vi "Find Average Center.vi"(5 "Position":i32, 7 "Tray Number":i32, 9 "XYZTheta":dbl[](array[numeric]), 11 "Gantry In":refnum<k24>) -> (1 "XYZTheta":dbl[](array[numeric]) format="%.6g", 3 "Gantry Out":refnum<k24>)   [LabVIEW 2019, in "Component Tray.lvclass"]
uses:
  Component Tray.lvclass
  Find Component.ctl
  Controller/Camera/Machine Vision.ctl
  C:/Program Files (x86)/Aerotech/A3200/LabVIEW/2010/Bin/Aerotech.A3200.dll
  Program Files (x86)/Aerotech/A3200/LabVIEW/2010/Bin/Aerotech.A3200.dll
  Controller/Camera/Image processing.ctl
  Controller/Camera/Camera settings.ctl
  Controller/Camera/Material.ctl
  Controller/Camera/Edmund Optics/Edmund Optics.lvclass
  C:/Users/HEP/Documents/Aerotech gantry/UCSB-Gantry-master-main/V5/Classes/Controller/Camera/Camera.lvclass
  Controller/Motion/A3200/A3200.lvclass
  Controller/Camera/Camera.lvclass
panel:
  in  "Material":T1
  out "All fiducials recorded":bool
  in  "Override presets":bool
  in  "Camera settings":T2={"Gamma"=1.6, "Gain"=0, "Sharpness"=0, "Contrast"=0.0, "Exposure"=0.0078125} {"Exposure" min=0.000244140625 max=0.5 scale=0.0002..0.5; "Contrast" min=0.0 max=1.0 scale=0.001..1.0; "Sharpness" min=0 max=2 step=1 scale=0.0..2.0; "Gain" min=0 max=100 step=1 scale=0.1..100.0; "Gamma" min=0.01 max=10.0 scale=0.01..10.0}
  in  "Image processing":T3={"Brightness"=128.0, "Contrast"=45.0, "Gamma"=1.0471123} {"Brightness" scale=0.0..400.0; "Contrast" scale=0.0..90.0; "Gamma" scale=0.005..5.0}
  in  "Machine Vision":T4
  out "Gantry":dbl[](array[numeric])
  out "Sum":dbl[](array[numeric])
  out "BR XY":dbl[](array[numeric]) format="%.6g"
  out "TR XY":dbl[](array[numeric]) format="%.6g"
  out "BL XY":dbl[](array[numeric]) format="%.6g"
  out "TL XY":dbl[](array[numeric]) format="%.6g"
  in  "Record Top Right":bool
  in  "Record Bottom Right":bool
  in  "Record Bottom Left":bool
  in  "Record Top Left":bool
  in  "Go to Bottom Right":bool
  in  "Go to Top Right":bool
  in  "Go to Bottom Left":bool
  in  "Go to Top Left":bool
  in  "Joystick":bool
  out "Camera":dbl[](array[numeric])
  in  "Go to Center":bool
  in  "Component":T5
  in  "Stop Program":bool
  out "Image":T6(plugin-control)
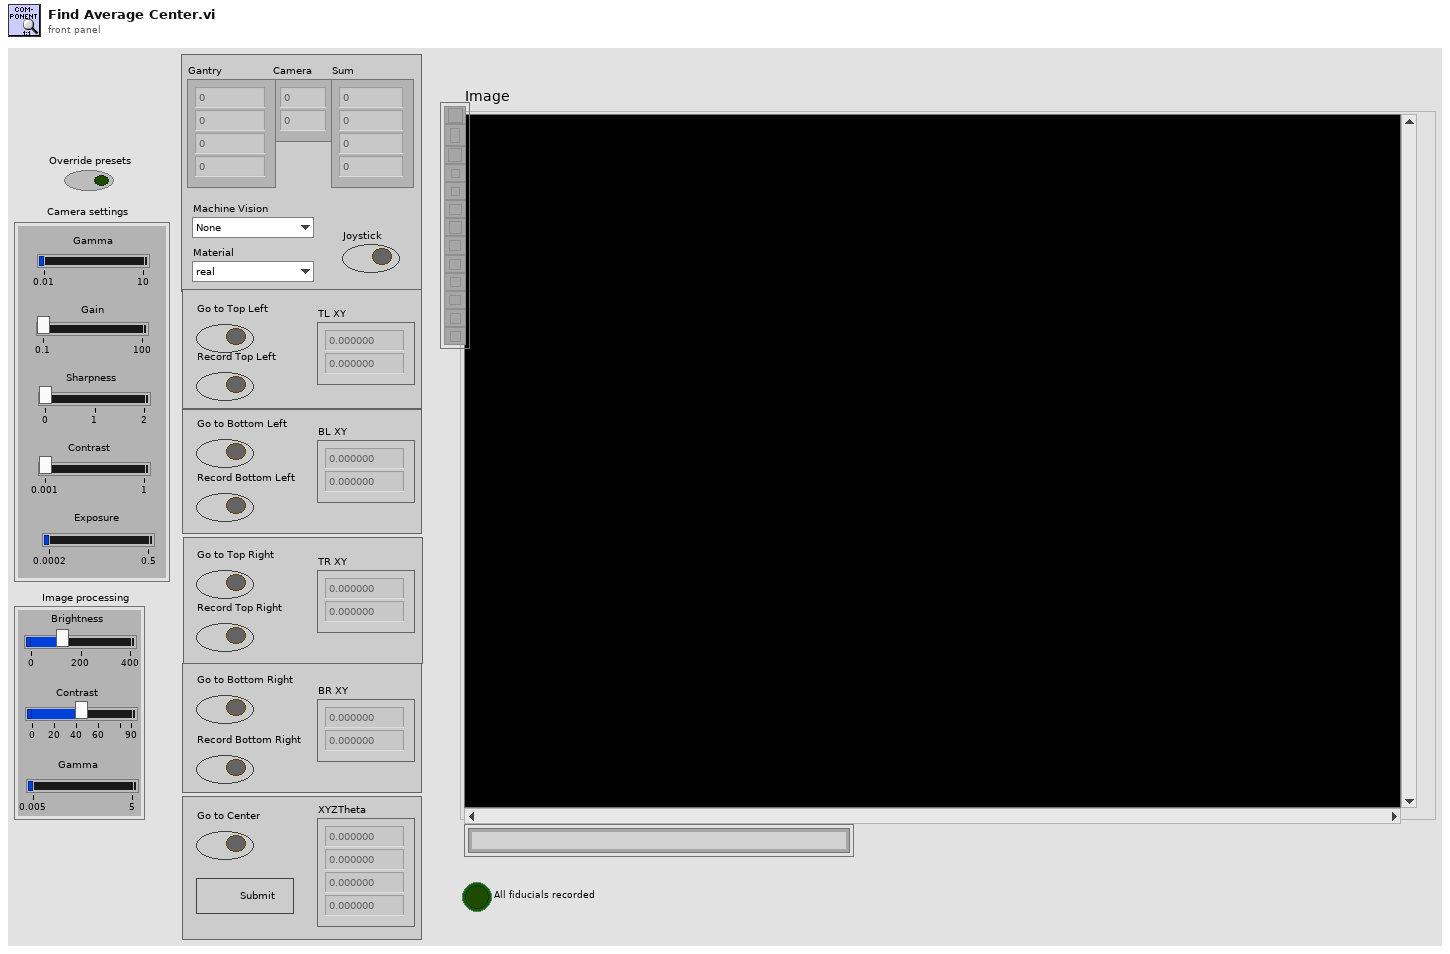
[diagram p1: front panel]
types:
  T1 = typedef "Camera.lvclass/Material.ctl" = enum16{"real", "dummy", "PETG"}
  T2 = typedef "Camera.lvclass/Camera settings.ctl" = cluster{"Gamma":dbl, "Gain":i64, "Sharpness":i64, "Contrast":dbl, "Exposure":dbl}
  T3 = typedef "Camera.lvclass/Image processing.ctl" = cluster{"Brightness":sgl, "Contrast":sgl, "Gamma":sgl}
  T4 = typedef "Camera.lvclass/Machine Vision.ctl" = enum16{"None", "Tray Fiducials", "HPK Silicon", "Hexaboard", "Corner (TL, BR)", "Corner (BL, TR)", "sensor TL", "sensor BL", "sensor TR", "sensor BR", "hexaboard TL", "hexaboard BL", "hexaboard TR", "hexaboard BR"}
  T5 = typedef "Component Tray.lvclass/Find Component.ctl" = cluster{"New Fiducials":dbl[], "Past Fiducials":dbl[], "XYZTheta":dbl[], "Fiducials Path":path, "Position":i32}
  T6 = typedef "IMAQ Image.ctl" = refnum<image>
  T7 = typedef "File Paths.ctl" = cluster{"Glue Pattern Folder":path, "Carrier Tray Folder":path, "Pick Up Tool Fixture Folder":path, "Components Folder":path, "Bellows Tool Offset.txt":path, "Pick Up Tool Offset.txt":path, "Dispense Tip Offset.txt":path, "Log Files":path}
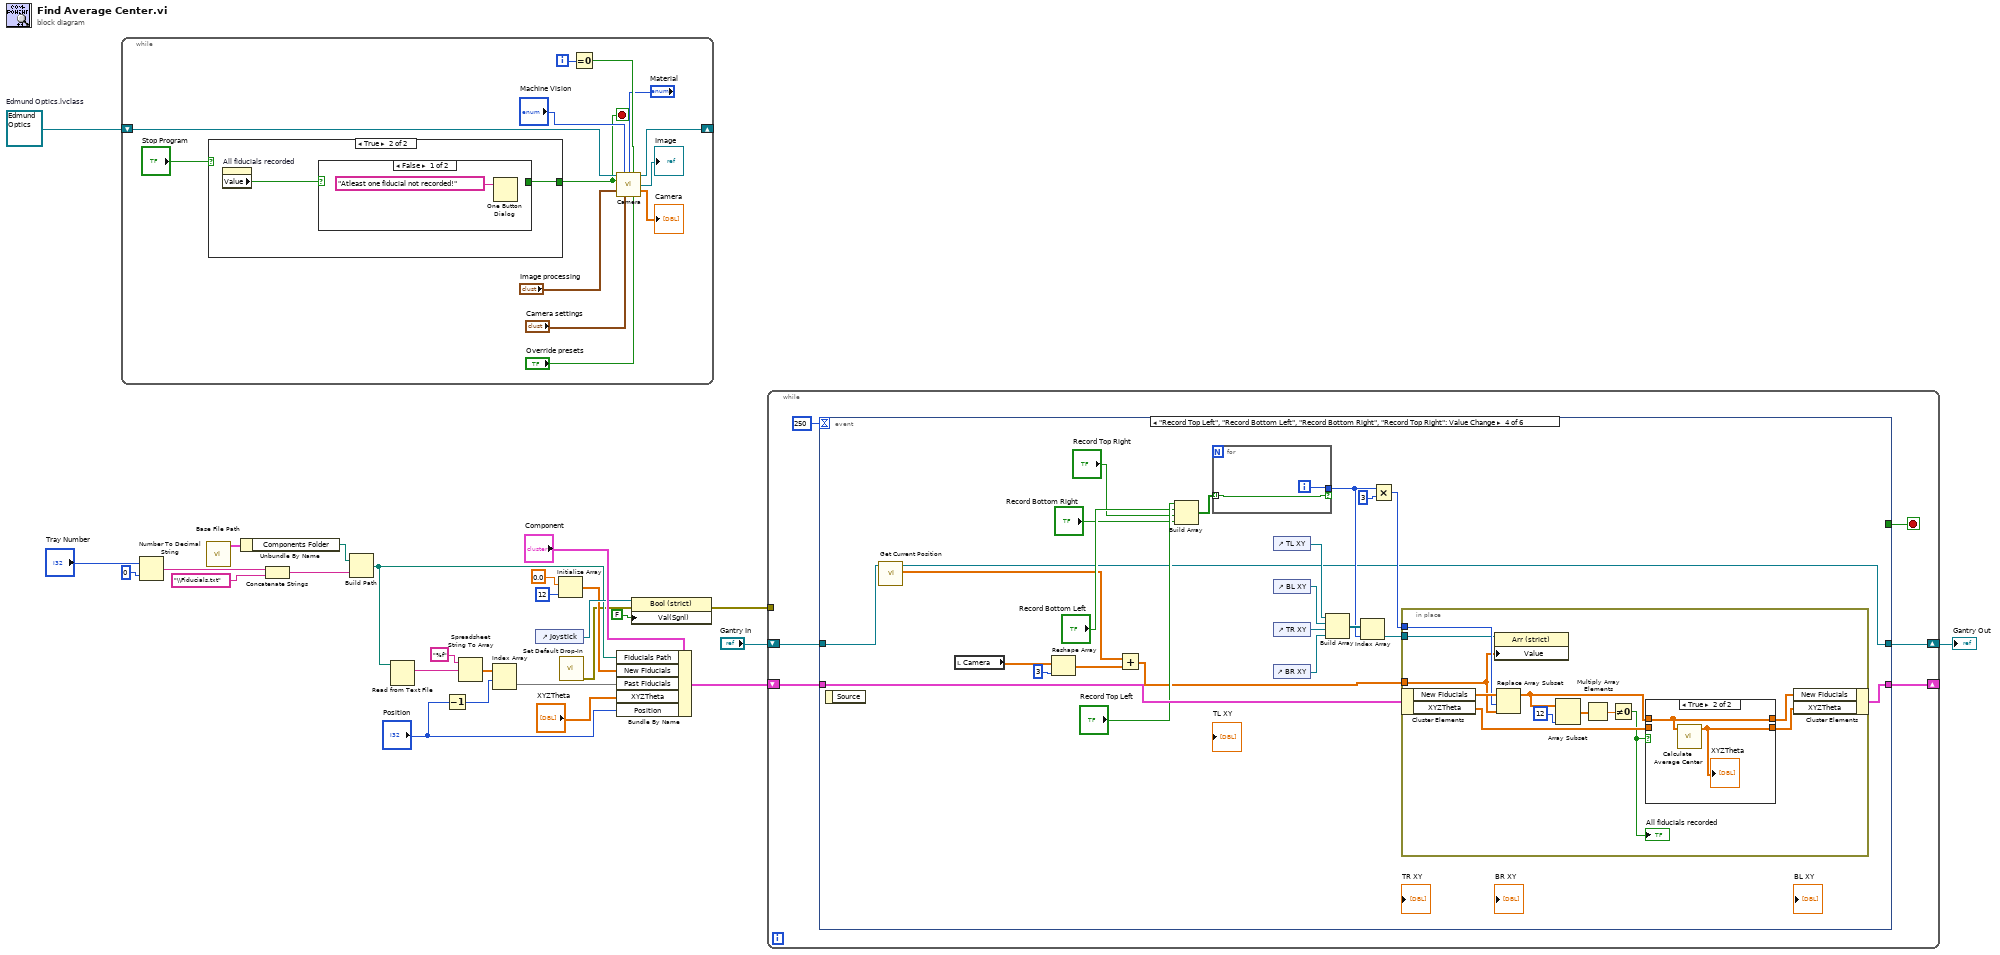
[diagram p0: block diagram]
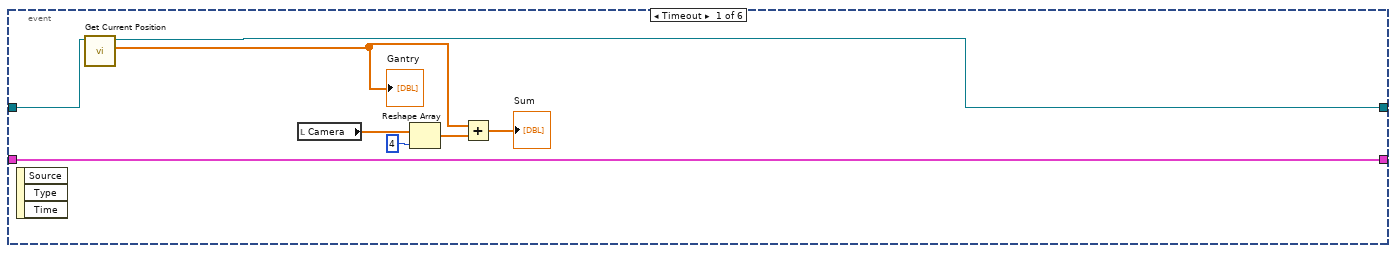
[diagram p2: hidden frame]
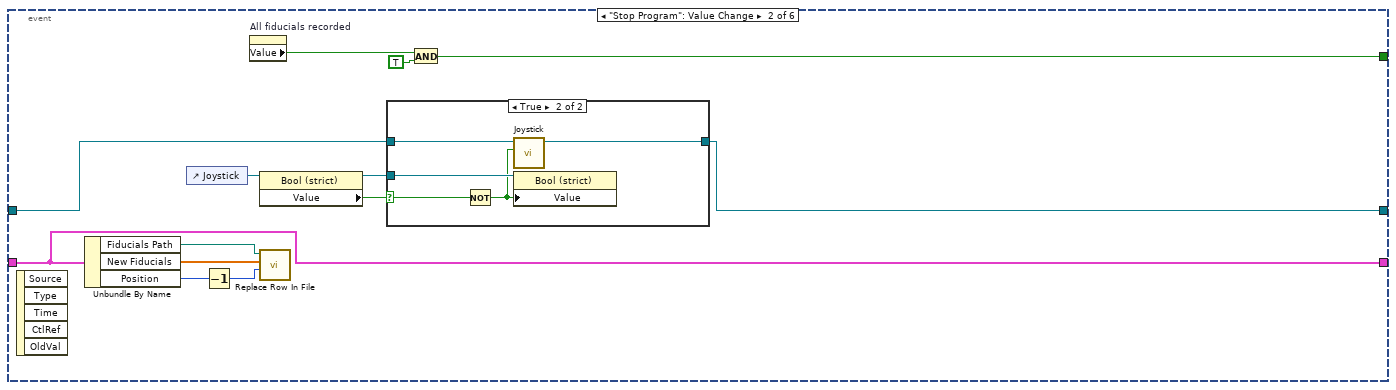
[diagram p3: hidden frame]
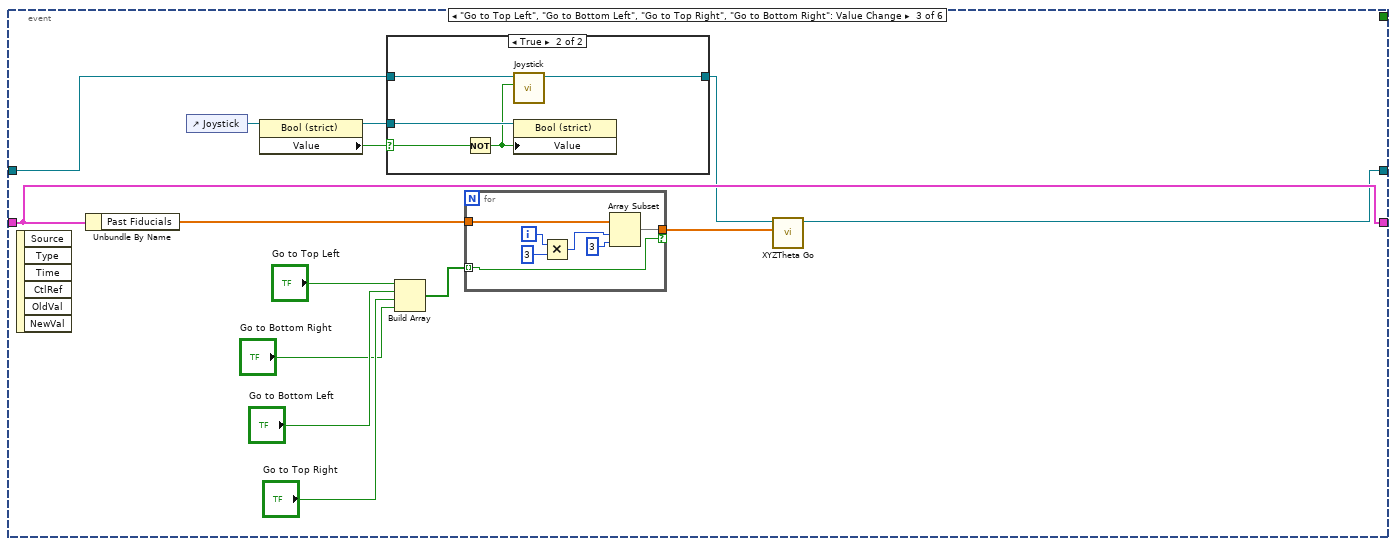
[diagram p5: hidden frame]
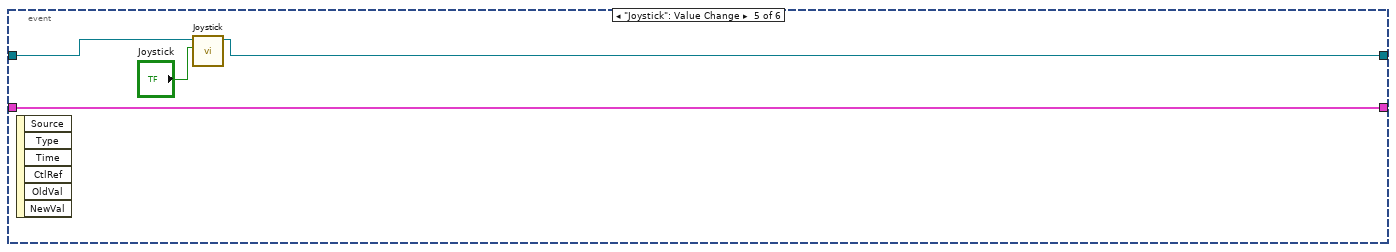
[diagram p8: hidden frame]
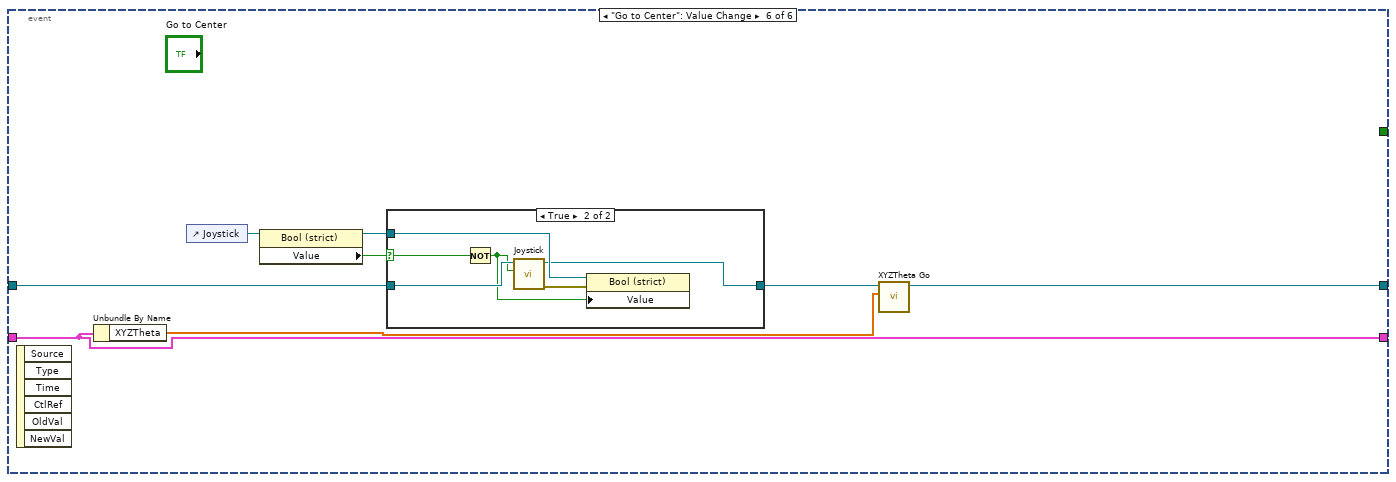
[diagram p9: hidden frame]
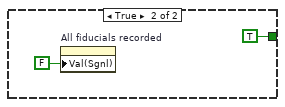
[diagram p12: hidden frame]
diagram:
  w22 = refnum<class "Edmund Optics.lvclass"> refnum  # Edmund Optics.lvclass
  n1 = while {
    shift-right: [w36] -> _
    shift-left: w22 -> [w40]
    i -> [w32]
    stop <- w29 stop-if-true
    n2 = case shown="True" "Stop Program" {
      tunnel: [_ w42] -> w29
      frame False {
      }
      frame True {
        n3 = property on="All fiducials recorded" class="Bool (strict)"() -> ("Value"=w41:bool)  [unwired: 2 in, 2 out]
        n4 = case shown="False" w41 {
          tunnel: [_ TRUE] -> w42
          frame False {
            n5 = One Button Dialog(message="Atleast one fiducial not recorded!") -> ()  [unwired: 1 in, 1 out]
          }
          frame True {
            n6 = property on="All fiducials recorded" class="Bool (strict)"("Val(Sgnl)"=FALSE) -> ()  [unwired: 2 in, 2 out]
          }
        }
      }
    }
    n7 = Equal To 0?(x=w32) -> (x = 0?=w31:bool)
    n8 = call "Camera.vi"("Camera in"=w40, "Machine Vision"="Machine Vision", "Material"="Material", "Loop 0"=w31, "Stop"=w29, "BCG Image Processing"="Image processing", "Camera settings"="Camera settings", "Override presets"="Override presets") -> ("Camera out"=w36:refnum<class "Edmund Optics.lvclass">, "Image"=→"Image":T6, "Camera"=→"Camera":dbl[])  [unwired: 4 in, 1 out]
  }
  n9 = Number To Decimal String(number="Tray Number", width (-)=i16 0) -> (decimal integer string=w16:string)
  n10 = call "Base File Path.vi"() -> ("Paths Out"=w13:T7)  [unwired: 11 in]
  n11 = Unbundle By Name(w13) -> ("Components Folder"=w15:path)
  n12 = Concatenate Strings(w16, "\\Fiducials.txt" ("string")) -> (w18:string)
  n13 = Build Path(base path=w15, name or relative path=w18) -> (appended path=w7:path)
  n14 = Read from Text File(file (use dialog)=w7) -> (text=w19:string)  [unwired: 3 in, 3 out]
  n15 = Decrement(x="Position") -> (x-1=w4:i32)
  n16 = Spreadsheet String To Array(format string="%f", spreadsheet string=w19) -> (array=w21:dbl[][])  [unwired: 2 in]
  n17 = Index Array(array=w21, index (row)=w4) -> (element=w11:dbl[])  [unwired: 1 in]
  n18 = control-ref of="Joystick"() -> (w25:refnum<vi>)
  n19 = Initialize Array(0.0 ("element"), 12 ("dimension size")) -> (w10:dbl[])
  n20 = call "Set Default Drop-In.vi"() -> ("error out"=w3:errorcluster)  [unwired: 11 in]
  n21 = Bundle By Name(cluster="Component", "Fiducials Path"=w7, "New Fiducials"=w10, "Past Fiducials"=w11, "XYZTheta"="XYZTheta", "Position"="Position") -> (w26:T5)
  n22 = property class="Bool (strict)"(reference=w25, error in=w3, "Val(Sgnl)"=FALSE) -> (error out=w23:errorcluster)  [unwired: 1 out]
  n23 = while {
    shift-right: [w49] -> _
    shift-left: w26 -> [w50]
    tunnel: w23 -> [_]
    shift-right: [w46] -> w1
    shift-left: "Gantry In" -> [w47]
    stop <- w51 stop-if-true
    n24 = event shown="[3] \"Record Top Left\", \"Record Bottom Left\", \"Record Bottom Right\", \"Record Top Right\": Value Change" {
      selector: _ -> [_ _ _ _ _ _]
      dyn-events: _ -> [_ _ _ _ _ _]
      timeout: 250 -> [_ _ _ _ _ _]
      tunnel: [_ w61 _ _ _ _] -> w51
      tunnel: w50 -> [w58 w68 w85 w128 w150 w157]
      tunnel: [w58 w68 w85 w127 w150 w157] -> w49
      tunnel: w47 -> [w54 w69 w82 w108 w149 w153]
      tunnel: [w53 w63 w79 w106 w147 w151] -> w46
      event Timeout {
        n25 = event-data() -> ()  [unwired: 1 in, 3 out]
        n26 = call "Get Current Position.vi"("Gantry In"=w54) -> ("XYZTheta Out"=w52:dbl[], "Gantry Out"=w53:refnum<k24>)  [unwired: 8 in, 1 out]
        "Gantry" <- w52
        n27 = local read "Camera"() -> (w57:dbl[])
        n28 = Reshape Array(w57, 4 ("dimension size")) -> (w55:dbl[])
        n29 = Add(x=w52, y=w55) -> (x+y=→"Sum":dbl[])
      }
      event "Stop Program": Value Change {
        n30 = event-data() -> ()  [unwired: 1 in, 5 out]
        n31 = Unbundle By Name(w68) -> ("Fiducials Path"=w66:path, "New Fiducials"=w67:dbl[], "Position"=w65:i32)
        n32 = control-ref of="Joystick"() -> (w70:refnum<vi>)
        n33 = Decrement(x=w65) -> (x-1=w64:i32)
        n34 = property on="All fiducials recorded" class="Bool (strict)"() -> ("Value"=w60:bool)  [unwired: 2 in, 2 out]
        n35 = property class="Bool (strict)"(reference=w70) -> (reference out=w71:refnum<vi>, "Value"=w72:bool)  [unwired: 1 in, 1 out]
        n36 = call "Replace Row In File.vi"("Index"=w64, "Insert Array"=w67, "Path"=w66) -> ()  [unwired: 8 in, 1 out]
        n37 = case shown="True" w72 {
          selector: w72 -> [_ w78]
          tunnel: w69 -> [w73 w76]
          tunnel: [w73 w75] -> w63
          tunnel: w71 -> [_ w77]
          frame False {
          }
          frame True {
            n38 = Not(x=w78) -> (.not. x?=w74:bool)
            n39 = call "Joystick.vi"("Joystick"=w74, "Gantry In"=w76) -> ("Gantry Out"=w75:refnum<k24>)  [unwired: 8 in, 1 out]
            n40 = property class="Bool (strict)"(reference=w77, "Value"=w74) -> ()  [unwired: 1 in, 2 out]
          }
        }
        n41 = And(x=w60, y=TRUE) -> (x .and. y?=w61:bool)
      }
      event "Go to Top Left", "Go to Bottom Left", "Go to Top Right", "Go to Bottom Right": Value Change {
        n42 = event-data() -> ()  [unwired: 1 in, 6 out]
        n43 = Unbundle By Name(w85) -> ("Past Fiducials"=w87:dbl[])
        n44 = control-ref of="Joystick"() -> (w80:refnum<vi>)
        n45 = property class="Bool (strict)"(reference=w80) -> (reference out=w83:refnum<vi>, "Value"=w84:bool)  [unwired: 1 in, 1 out]
        n46 = case shown="True" w84 {
          selector: w84 -> [_ w98]
          tunnel: w82 -> [w93 w96]
          tunnel: [w93 w94] -> w81
          tunnel: w83 -> [_ w97]
          frame False {
          }
          frame True {
            n47 = Not(x=w98) -> (.not. x?=w95:bool)
            n48 = call "Joystick.vi"("Joystick"=w95, "Gantry In"=w96) -> ("Gantry Out"=w94:refnum<k24>)  [unwired: 8 in, 1 out]
            n49 = property class="Bool (strict)"(reference=w97, "Value"=w95) -> ()  [unwired: 1 in, 2 out]
          }
        }
        n50 = Build Array("Go to Top Left", "Go to Bottom Left", "Go to Top Right", "Go to Bottom Right") -> (w88:bool[])
        n51 = for {
          tunnel: w88 -> [w105] mode=indexing
          tunnel: w87 -> [w104]
          tunnel: [w99] -> w86 if=w105
          i -> [w102]
          n52 = Multiply(x=w102, y=3) -> (x*y=w100:i32)
          n53 = Array Subset(array=w104, index=w100, length=3) -> (w99:dbl[])
        }
        n54 = call "XYZTheta Go.vi"("XYZTheta In"=w86, "Gantry In"=w81) -> ("Gantry Out"=w79:refnum<k24>)  [unwired: 7 in, 2 out]
      }
      event "Record Top Left", "Record Bottom Left", "Record Bottom Right", "Record Top Right": Value Change {
        n55 = event-data() -> ()  [unwired: 1 in, 1 out]
        n56 = call "Get Current Position.vi"("Gantry In"=w108) -> ("XYZTheta Out"=w107:dbl[], "Gantry Out"=w106:refnum<k24>)  [unwired: 8 in, 1 out]
        n57 = local read "Camera"() -> (w111:dbl[])
        n58 = Reshape Array(w111, 3 ("dimension size")) -> (w110:dbl[])
        n59 = Add(x=w107, y=w110) -> (x+y=w109:dbl[])
        n60 = Build Array("Record Top Left", "Record Bottom Left", "Record Top Right", "Record Bottom Right") -> (w122:bool[])
        n61 = for {
          tunnel: w122 -> [w129] mode=indexing
          tunnel: [w130] -> w114 if=w129
          i -> [w130]
        }
        n62 = control-ref of="TL XY"() -> (w121:refnum<vi>)
        n63 = control-ref of="BL XY"() -> (w120:refnum<vi>)
        n64 = control-ref of="TR XY"() -> (w119:refnum<vi>)
        n65 = control-ref of="BR XY"() -> (w118:refnum<vi>)
        n66 = Build Array(w121, w120, w119, w118) -> (w117:refnum<vi>[])
        n67 = Index Array(array=w117, index=w114) -> (element=w116:refnum<vi>)
        n68 = Multiply(x=w114, y=3) -> (x*y=w112:i32)
        n69 = in-place {
          in-place-border: w112 -> [w140]
          in-place-border: w116 -> [w138]
          in-place-border: w109 -> [w136]
          n70 = in-place-cluster #1(w128) -> ("New Fiducials"=w141:dbl[], "XYZTheta"=w137:dbl[])
          n71 = property class="Arr (strict)"(reference=w138, "Value"=w136) -> ()  [unwired: 1 in, 2 out]
          n72 = Replace Array Subset(array=w141, new element=w136, index=w140) -> (w135:dbl[])
          n73 = Array Subset(array=w135, length=12) -> (w133:dbl[])  [unwired: 1 in]
          n74 = Multiply Array Elements(1:w133) -> (0:w132:dbl)
          n75 = Not Equal To 0?(x=w132) -> (x != 0?=w131:bool)
          "All fiducials recorded" <- w131
          n76 = case shown="True" w131 {
            tunnel: [w143 w145] -> w142
            tunnel: w135 -> [w144 w146]
            tunnel: [w144 w146] -> w139
            tunnel: w137 -> [w143 _]
            frame False {
            }
            frame True {
              n77 = call "Calculate Average Center.vi"("Gantry Fiducials"=w146) -> ("XYZTheta"=w145:dbl[])  [unwired: 10 in]
              "XYZTheta" <- w145
            }
          }
          n78 = in-place-cluster #1("New Fiducials"=w139, "XYZTheta"=w142) -> (w127:T5)
        }
      }
      event "Joystick": Value Change {
        n79 = event-data() -> ()  [unwired: 1 in, 6 out]
        n80 = call "Joystick.vi"("Joystick"="Joystick", "Gantry In"=w149) -> ("Gantry Out"=w147:refnum<k24>)  [unwired: 8 in, 1 out]
      }
      event "Go to Center": Value Change {
        n81 = event-data() -> ()  [unwired: 1 in, 6 out]
        n82 = Unbundle By Name(w157) -> ("XYZTheta"=w158:dbl[])
        n83 = control-ref of="Joystick"() -> (w154:refnum<vi>)
        n84 = property class="Bool (strict)"(reference=w154) -> (reference out=w155:refnum<vi>, "Value"=w156:bool)  [unwired: 1 in, 1 out]
        n85 = case shown="True" w156 {
          selector: w156 -> [_ w165]
          tunnel: w153 -> [w159 w162]
          tunnel: [w159 w161] -> w152
          tunnel: w155 -> [_ w164]
          frame False {
          }
          frame True {
            n86 = Not(x=w165) -> (.not. x?=w160:bool)
            n87 = call "Joystick.vi"("Joystick"=w160, "Gantry In"=w162) -> ("error out"=w163:errorcluster, "Gantry Out"=w161:refnum<k24>)  [unwired: 8 in]
            n88 = property class="Bool (strict)"(reference=w164, error in=w163, "Value"=w160) -> ()  [unwired: 2 out]
          }
        }
        n89 = call "XYZTheta Go.vi"("XYZTheta In"=w158, "Gantry In"=w152) -> ("Gantry Out"=w151:refnum<k24>)  [unwired: 7 in, 2 out]
      }
    }
  }
  "Gantry Out" <- w1
